vi "Write ADS State.vi"(8 "error in (no error)":errorcluster, 10 "ADS State":i16(ring) items=["Invalid", "Idle", "Reset", "Init", "Start", "Run", "Stop", "SaveConfig", "LoadConfig", "PowerFailure", "PowerGood", "Error", "Shutdown", "Suspend", "Resume", "Config", "Reconfig", "Stopping, Maxstates", "Incompatible", "Exception"], 11 "TwinCAT ADS in":refnum<class "TwinCAT ADS.lvclass">) -> (0 "error out":errorcluster, 3 "TwinCAT ADS out":refnum<class "TwinCAT ADS.lvclass">)   [LabVIEW 2018, in "TwinCAT ADS.lvclass"]
uses:
  TwinCAT ADS.lvclass
  TwinCAT ADS.lvclass/TwinCAT ADS.ctl
  TwinCAT.Ads
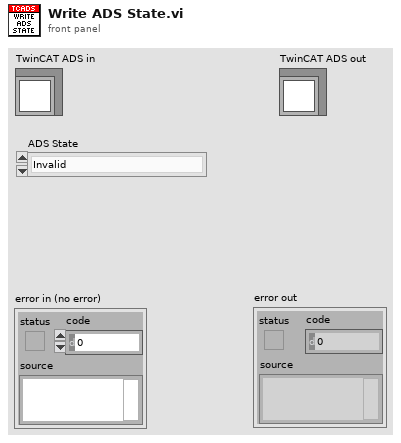
[diagram p1: front panel]
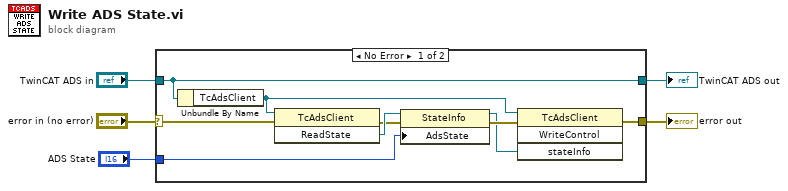
[diagram p0: block diagram]
diagram:
  n1 = case shown="No Error" "error in (no error)" {
    selector: "error in (no error)" -> [w7 w16]
    tunnel: [w11 w16] -> w4
    tunnel: [w14 w15] -> w2
    tunnel: "TwinCAT ADS in" -> [w14 w15]
    tunnel: "ADS State" -> [w6 _]
    frame No Error {
      n2 = Unbundle By Name(w14) -> ("TcAdsClient"=w9:refnum<k24>)
      n3 = invoke class="TcAdsClient" method="ReadState"(reference=w9, error in=w7) -> (error out=w8:errorcluster, "ReadState"=w10:refnum<k24>)  [unwired: 1 in, 1 out]
      n4 = property class="StateInfo"(reference=w10, error in=w8, "AdsState"=w6) -> (reference out=w12:refnum<k24>, error out=w13:errorcluster)
      n5 = invoke class="TcAdsClient" method="WriteControl"(reference=w9, error in=w13, "stateInfo"=w12) -> (error out=w11:errorcluster)  [unwired: 1 in, 3 out]
    }
    frame Error {
    }
  }
  "error out" <- w4
  "TwinCAT ADS out" <- w2
